vi "Coord window-Load setup.vi"(8 "error in (no error)":errorcluster) -> (0 "error out":errorcluster)   [LabVIEW 2013]
uses:
  Typedefs/Save-Load enum.ctl
  Visualisation/Functional Imaging Viewer/Typedefs/Get-Set-Clear Control.ctl
  Globals/Coord window-Globals.vi
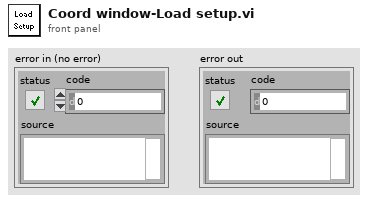
[diagram p1: front panel]
types:
  T1 = typedef "Save-Load enum.ctl" = enum16{"Save to file", "Load from file", "Compare from file"}
  T2 = typedef "Get-Set-Clear Control.ctl" = enum16{"Get", "Set", "Clear"}
  T3 = typedef "Coordinate list window refs.ctl" = cluster{"Window Name (i.e. Key)":string, "menu reference":refnum<k9>, "VI's reference":refnum<vi>, "Pane 1":refnum<vi>, "Pane 2":refnum<vi>, "Coord Listbox":refnum<vi>, "File name":refnum<vi>, "Picture Map":refnum<vi>, "Stage XYZ Position ind.":refnum<vi>}
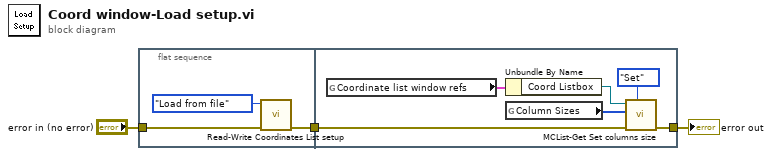
[diagram p0: block diagram]
diagram:
  n1 = flat-sequence {
    tunnel: [w6] -> w3
    tunnel: "error in (no error)" -> [w5]
    tunnel: [w9] -> w1
    tunnel: w3 -> [w12]
    frame #0 {
      n2 = call "Read-Write Coordinates List setup.vi"("error in"=w5, "Function"=Save-Load_enum."Load from file") -> ("error out"=w6:errorcluster)  [unwired: 9 in]
    }
    frame #1 {
      n3 = global read "Coord window-Globals.vi" "Coordinate list window refs"() -> (w8:T3)
      n4 = Unbundle By Name(w8) -> ("Coord Listbox"=w7:refnum<vi>)
      n5 = global read "Coord window-Globals.vi" "Column Sizes"() -> (w10:u32[])
      n6 = call "MCList-Get Set columns size.vi"("Function"=Get-Set-Clear_Control."Set", "error in (no error)"=w12, "Column Sizes"=w10, "Listbox ref"=w7) -> ("Error out"=w9:errorcluster)  [unwired: 6 in, 1 out]
    }
  }
  "error out" <- w1
